vi "Finish.vi"   [LabVIEW 2016]
doc: "This VI is called just before exiting. It is expected to close I/O refnum, save collected data, etc."
uses:
  <vilib>/Rock Robotics/WPI/Utilities/WPI_GetSetVariantRefNum.vi
  <vilib>/Rock Robotics/WPI/Ultrasonic/WPI_SonarMB1010AnalogRefNum Registry Get.vi
  <vilib>/Rock Robotics/WPI/Ultrasonic/WPI_SonarMB1010AnalogClose.vi
types:
  T1 = typedef "WPI_MotorControlDeviceRef.ctl" = cluster{"DeviceStatus":errorcluster, "Type":T2, "PWM":cluster{"PWM Channel":T3, "DeadBand":T4}, "CAN":cluster{"Device Number":u8, "SetOutput VI Ref":variant, "GetOutput VI Ref":variant, "Enable VI Ref":variant, "Disable VI Ref":variant, "Data":variant}, "Invert":bool}
  T2 = typedef "WPI_MotorControlType.ctl" = enum16{"PWM", "CAN"}
  T3 = typedef "FPGA_DIOPWMChannel.ctl" = enum8{"PWM 0", "PWM 1", "PWM 2", "PWM 3", "PWM 4", "PWM 5", "PWM 6", "PWM 7", "PWM 8", "PWM 9", "PWM MXP 0", "PWM MXP 1", "PWM MXP 2", "PWM MXP 3", "PWM MXP 4", "PWM MXP 5", "PWM MXP 6", "PWM MXP 7", "PWM MXP 8", "PWM MXP 9", "Invalid"}
  T4 = typedef "WPI_PWMDeadband.ctl" = cluster{"Name":string, "maxPositivePwm":i32, "minPositivePwm":i32, "centerPwm":i32, "maxNegativePwm":i32, "minNegativePwm":i32, "angularRange":u16}
  T5 = typedef "WPI_SwitchDevRef.ctl" = cluster{"DevStatus":errorcluster, "DIO Channel":T6, "CntIndex":T7, "Normally Closed":bool}
  T6 = typedef "FPGA_DIOChannel.ctl" = enum8{"DIO 0", "DIO 1", "DIO 2", "DIO 3", "DIO 4", "DIO 5", "DIO 6", "DIO 7", "DIO 8", "DIO 9", "DIO MXP 0", "DIO MXP 1", "DIO MXP 2", "DIO MXP 3", "DIO MXP 4", "DIO MXP 5", "DIO MXP 6", "DIO MXP 7", "DIO MXP 8", "DIO MXP 9", "DIO MXP 10", "DIO MXP 11", "DIO MXP 12", "DIO MXP 13", "DIO MXP 14", "DIO MXP 15", "SPI Port CS1", "SPI Port CS2", "SPI Port CS3", "SPI Port MISO", "SPI Port MOSI", "Invalid"}
  T7 = typedef "FPGA_CounterCtrSystemIndex.ctl" = enum8{"Ctr 0", "Ctr 1", "Ctr 2", "Ctr 3", "Ctr 4", "Ctr 5", "Ctr 6", "Ctr 7", "Invalid"}
  T8 = typedef "WPI_SonarMB1010AnalogDeviceRef.ctl" = cluster{"AIDeviceRef":T9, "Scaling factor (V/in)":dbl, "Average Bits":u8}
  T9 = typedef "WPI_AnalogChannelDevRef.ctl" = cluster{"DevStatus":errorcluster, "Analog Channel":T10}
  T10 = typedef "FPGA_AIChannel.ctl" = enum8{"AI 0", "AI 1", "AI 2", "AI 3", "AI MXP 0", "AI MXP 1", "AI MXP 2", "AI MXP 3", "Invalid"}
  T11 = typedef "WPI_DigitalOutputDevRef.ctl" = cluster{"DIO Channel":T6, "DevStatus":errorcluster}
  T12 = typedef "WPI_JoystickDevRef.ctl" = cluster{"Device":T13}
  T13 = typedef "WPI_JoystickDeviceEnum.ctl" = enum16{"USB 0", "USB 1", "USB 2", "USB 3", "USB 4", "USB 5"}
  T14 = typedef "WPI_RobotDriveDevRef.ctl" = cluster{"DevStatus":errorcluster, "Motors[]":T1[], "Square Inputs":bool, "Max Output":dbl}
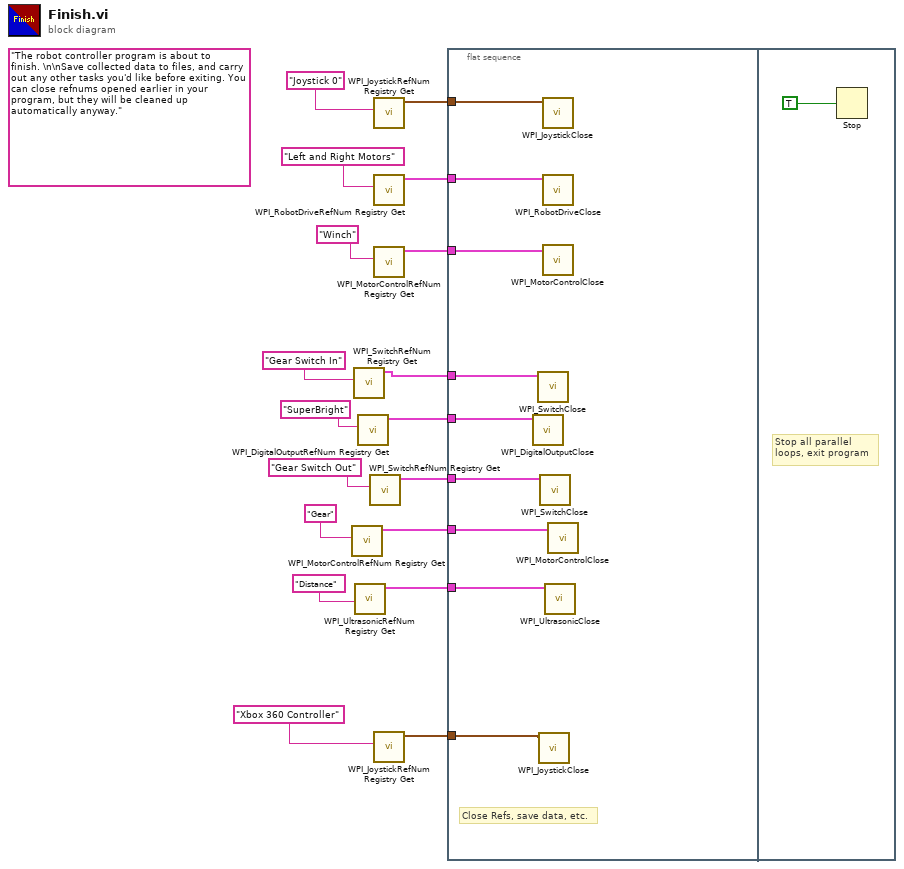
[diagram p0: block diagram]
diagram:
  (unwired) "The robot controller program is about to finish. \n\nSave collected data to files, and carry out any other tasks you'd like before exiting. You can close refnums opened earlier in your program, but they will be cleaned up automatically anyway."
  n1 = call <vilib>:"WPI_MotorControlRefNum Registry Get.vi"("refnum name"="Gear") -> ("MotorControlDevRef"=w9:T1)  [unwired: 9 in, 1 out]
  n2 = call <vilib>:"WPI_SwitchRefNum Registry Get.vi"("refnum name"="Gear Switch In") -> ("SwitchDevRef"=w4:T5)  [unwired: 9 in, 1 out]
  n3 = call-poly <vilib>:"WPI_UltrasonicRefNum Registry Get.vi"("refnum name"="Distance") -> ("SonarMB1010AnalogDevRef"=w7:T8)  [unwired: 9 in, 1 out]
  n4 = call <vilib>:"WPI_DigitalOutputRefNum Registry Get.vi"("refnum name"="SuperBright") -> ("DigitalOutputDevRef"=w2:T11)  [unwired: 9 in, 1 out]
  n5 = call <vilib>:"WPI_SwitchRefNum Registry Get.vi"("refnum name"="Gear Switch Out") -> ("SwitchDevRef"=w11:T5)  [unwired: 9 in, 1 out]
  n6 = call <vilib>:"WPI_JoystickRefNum Registry Get.vi"("refnum name"="Joystick 0") -> ("JoystickDevRef"=w15:T12)  [unwired: 1 in, 9 out]
  n7 = call <vilib>:"WPI_RobotDriveRefNum Registry Get.vi"("refnum name"="Left and Right Motors") -> ("RobotDriveDevRef"=w16:T14)  [unwired: 1 in, 9 out]
  n8 = call <vilib>:"WPI_MotorControlRefNum Registry Get.vi"("refnum name"="Winch") -> ("MotorControlDevRef"=w13:T1)  [unwired: 9 in, 1 out]
  n9 = call <vilib>:"WPI_JoystickRefNum Registry Get.vi"("refnum name"="Xbox 360 Controller") -> ("JoystickDevRef"=w5:T12)  [unwired: 1 in, 9 out]
  n10 = flat-sequence {
    tunnel: w16 -> [w27]
    tunnel: w15 -> [w26]
    tunnel: w13 -> [w25]
    tunnel: w11 -> [w24]
    tunnel: w9 -> [w23]
    tunnel: w7 -> [w22]
    tunnel: w5 -> [w21]
    tunnel: w4 -> [w20]
    tunnel: w2 -> [w19]
    frame #0 {
      # "Close Refs, save data, etc."
      n11 = call <vilib>:"WPI_DigitalOutputClose.vi"("DigitalOutputDevRef"=w19) -> ()  [unwired: 10 in, 1 out]
      n12 = call <vilib>:"WPI_SwitchClose.vi"("SwitchDevRef"=w20) -> ()  [unwired: 10 in, 1 out]
      n13 = call <vilib>:"WPI_JoystickClose.vi"("JoystickDevRef"=w21) -> ()  [unwired: 11 out]
      n14 = call <vilib>:"WPI_SwitchClose.vi"("SwitchDevRef"=w24) -> ()  [unwired: 10 in, 1 out]
      n15 = call <vilib>:"WPI_JoystickClose.vi"("JoystickDevRef"=w26) -> ()  [unwired: 11 out]
      n16 = call <vilib>:"WPI_RobotDriveClose.vi"("RobotDriveDevRef"=w27) -> ()  [unwired: 1 in, 10 out]
      n17 = call <vilib>:"WPI_MotorControlClose.vi"("MotorControlDevRef"=w25) -> ()  [unwired: 10 in, 1 out]
      n18 = call-poly <vilib>:"WPI_UltrasonicClose.vi"("SonarMB1010AnalogDevRef"=w22) -> ()  [unwired: 10 in, 1 out]
      n19 = call <vilib>:"WPI_MotorControlClose.vi"("MotorControlDevRef"=w23) -> ()  [unwired: 10 in, 1 out]
    }
    frame #1 {
      # "Stop all parallel\nloops, exit program"
      n20 = Stop(stop? (T)=TRUE ("Quit")) -> ()
    }
  }
